vi "Do.vi"(8 "error in":errorcluster, 10 "Actor in":refnum<class "Actor.lvclass">, 11 "File Data Message":refnum<class "File Data Message.lvclass">) -> (0 "error out":errorcluster, 2 "Actor out":refnum<class "Actor.lvclass">)   [LabVIEW 2017, in "File Library.lvlib" / "File Data Message.lvclass"]
doc: "(<B>Filename</B>: Actor Framework.lvlib:Message.lvclass:Do.vi)\n\nDefines what a message does when it is received by an actor. Generally, a message instructs an actor to invoke one of its methods. By default, this method does nothing. A child class must override it to define behavior. Create a child class by using the Actor Framework Message Maker dialog box."
uses:
  File Data Message.lvclass
  <vilib>/ActorFramework/Actor/Actor.lvclass
  File Actor.lvclass
  C:/Program Files (x86)/National Instruments/LabVIEW 2017/vi.lib/MSR Consulting, LLC/General Reuse/SuperActor/SuperActor.lvclass
  C:/Program Files (x86)/National Instruments/LabVIEW 2017/vi.lib/ActorFramework/Actor/Actor.lvclass
  <vilib>/MSR Consulting, LLC/General Reuse/SuperActor/SuperActor.lvclass/SuperActor.ctl
  File Actor.lvclass/File Actor.ctl
  <vilib>/MSR Consulting, LLC/General Reuse/SuperActor/Read Log Session.vi
  Read Exe File Write.vi
  Read Exe Write.vi
  Abstract/Exe Write/Exe Write.lvclass
  C:/Program Files (x86)/National Instruments/LabVIEW 2017/vi.lib/MSR Consulting, LLC/General Reuse/Command/Command.lvclass
  <vilib>/MSR Consulting, LLC/General Reuse/Command/Command.lvclass
  <vilib>/MSR Consulting, LLC/General Reuse/Session APIs/_Session Fwk/Session - Root.lvclass
  <vilib>/MSR Consulting, LLC/General Reuse/Session APIs/Session Log/System Log.lvclass
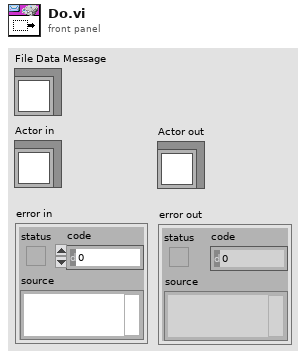
[diagram p1: front panel]
types:
  T1 = typedef "Session - Root.lvclass/Session Handle.ctl" = refnum<data-value>
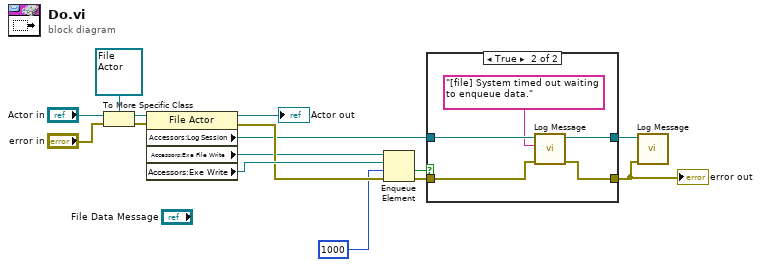
[diagram p0: block diagram]
diagram:
  n1 = To More Specific Class(target class=refnum<class "File Actor.lvclass"> refnum ("File Library.lvlib:File Actor"), reference="Actor in", error in="error in") -> (specific class reference=w12:refnum<class "File Actor.lvclass">, error out=w11:errorcluster)
  n2 = property class="File Actor"(reference=w12, error in=w11) -> (reference out=→"Actor out":refnum<class "File Actor.lvclass">, error out=w6:errorcluster, "Accessors:Log Session"=w1:T1, "Accessors:Exe File Write"=w2:refnum<queue>, "Accessors:Exe Write"=w7:refnum<class "Exe Write.lvclass">)
  n3 = Enqueue Element(queue=w2, element=w7, timeout in ms (-1)=1000, error in (no error)=w6) -> (timed out?=w4:bool, error out=w5:errorcluster)  [unwired: 1 out]
  n4 = case shown="True" w4 {
    tunnel: w5 -> [w17 w19]
    tunnel: w1 -> [w16 w22]
    tunnel: [w17 w18] -> w9
    tunnel: [w16 w20] -> w10
    frame False {
    }
    frame True {
      n5 = call <vilib>:"Log Message.vi"("error in"=w19, "MSG In"="[file] System timed out waiting to enqueue data.", "session in"=w22) -> ("error out"=w18:errorcluster, "session out"=w20:T1)  [unwired: 7 in]
    }
  }
  "error out" <- w9
  n6 = call <vilib>:"Log Message.vi"("error in"=w9, "session in"=w10) -> ()  [unwired: 8 in, 2 out]
